vi "Receiver_Example - 2 Channel - Experiment_1.vi"() -> ()   [LabVIEW 2022 SP3]
panel:
  out "Constellation Map 4":cluster{"Constellation":cdb[]}[](graph)
  out "No. Bits LP 2":dbl
  in  "Expected message 2 HP 3":string="Critical Dataaaaa\nCritical Dataaaaa\nCritical Dataaaaa\nCritical Dataaaaa\nCritical Dataaaaa"
  out "Inst. BER HP 3":dbl format="%#_4g"
  out "Acum. Err HP 3":dbl
  out "Acc. BER  HP 3":dbl format="%#_4g"
  out "No. Bits HP 3":dbl
  in  "Boolean 5":bool
  out "Expected message  HP  Detected 3":string="Critical Dataaaaa\nCritical Dataaaaa\nCritical Dataaaaa\nCritical Dataaaaa\nCritical Dataaaaa"
  out "Constellation Map 3":cdb[](graph)
  out "Iterations 2":i32
  in  "OFDM - 4QAM/16QAM":bool
  in  "Tab Control 2":enum32{"OFDM - 4QAM", "16QAM"}(tab)
  in  "Tab Control":enum32{"USRP Parameters", "Rx Info", "BER"}(tab)
  in  "USRP ControledParameters":T1={"Active Antenna"="RX2", "Gain (dB)"=10.0, "Carrier Frequency"=2400000000.0, "IQ Rate"=2000000.0, "Active channels"="0,1"} {"IQ Rate" format="%#_6p"; "Carrier Frequency" format="%#_6p"; "Gain (dB)" format="%#_6f"}
  in  "Device selection":refnum<k15>="RIO0"
  in  "Trigger level":dbl=0.005 format="%f"
  out "?":T2
  out "SIG valid?":bool
  out "Frequency offset":dbl
  out "Coerced Parameters":T3={"IQ Rate"=100000.0, "Carrier  Freq."=100000.0, "Gain"=0.0} {"Gain" format="%#_6f"; "Carrier  Freq." format="%#_6p"; "IQ Rate" format="%#_6p"}
  out "Error out":errorcluster
  out "Frequency offset 3":dbl
  out "SIG valid? 3":bool
  out "Error out 2":errorcluster
  out "?":T2
  in  "Boolean":bool
  in  "Expected message LP":string="Non Critical Data\nNon Critical Data\nNon Critical Data\nNon Critical Data\nNon Critical Data"
  in  "Record BER":bool
  in  "Refresh Button":bool
  out "Inst. BER LP":dbl format="%#_4g"
  out "No. Bits LP":dbl
  out "Acum. Err LP":dbl
  out "Acc. BER LP":dbl format="%#_4g"
  in  "Expected message 2 HP":string="Critical Dataaaaa\nCritical Dataaaaa\nCritical Dataaaaa\nCritical Dataaaaa\nCritical Dataaaaa"
  out "Inst. BER HP":dbl format="%#_4g"
  out "Acum. Err HP":dbl
  out "No. Bits HP":dbl
  out "Acc. BER  HP":dbl format="%#_4g"
  out "Expected message LP Detected":string="Non Critical Data\nNon Critical Data\nNon Critical Data\nNon Critical Data\nNon Critical Data"
  out "Expected message  HP  Detected":string="Critical Dataaaaa\nCritical Dataaaaa\nCritical Dataaaaa\nCritical Dataaaaa\nCritical Dataaaaa"
  in  "Boolean 2":bool
  out "Constellation Map":cdb[](graph)
  out "Low-Power Decoded Message":string
  out "High-Power Decoded Message":string
  out "Low-Power BER Graph":dbl(graph)
  out "High-Power BER Graph":dbl(graph)
  out "Low-Power Instantaneous BER Graph":u8(slide) scale=0.0..100.0
  out "High-Power Instantaneous BER Graph":u8(slide) scale=0.0..100.0
  in  "Low-Power Window Size":dbl=15.0 format="%#_6p"
  in  "High-Power Window Size":dbl=15.0 format="%#_6p"
  out "Reconstructed Image":T4(plugin-control)
  out "High-Power Decoded Message 3":string
  in  "High-Power Window Size 3":dbl=15.0 format="%#_6p"
  out "High-Power Instantaneous BER Graph 3":u8(slide) scale=0.0..100.0
  out "High-Power BER Graph 3":dbl(graph)
  out "Expected message  HP  Detected 2":string="Critical Dataaaaa\nCritical Dataaaaa\nCritical Dataaaaa\nCritical Dataaaaa\nCritical Dataaaaa"
  in  "Boolean 3":bool
  in  "High-Power Window Size 2":dbl=15.0 format="%#_6p"
  out "High-Power Instantaneous BER Graph 2":u8(slide) scale=0.0..100.0
  out "High-Power BER Graph 2":dbl(graph)
  out "No. Bits HP 2":dbl
  out "Acc. BER  HP 2":dbl format="%#_4g"
  out "Acum. Err HP 2":dbl
  out "Inst. BER HP 2":dbl format="%#_4g"
  in  "Expected message 2 HP 2":string="Critical Dataaaaa\nCritical Dataaaaa\nCritical Dataaaaa\nCritical Dataaaaa\nCritical Dataaaaa"
  out "High-Power Decoded Message 2":string
  in  "Record BER 2":bool
  out "Constellation Map 2":cdb[](graph)
  out "Frequency offset 2":dbl
  out "SIG valid? 2":bool
  in  "Refresh Button 2":bool
  out "Reconstructed Image":T4(plugin-control)
  out "Iterations":i32
  in  "error in (no error)":errorcluster
  # "OFDM Superposition Coded Receiver"
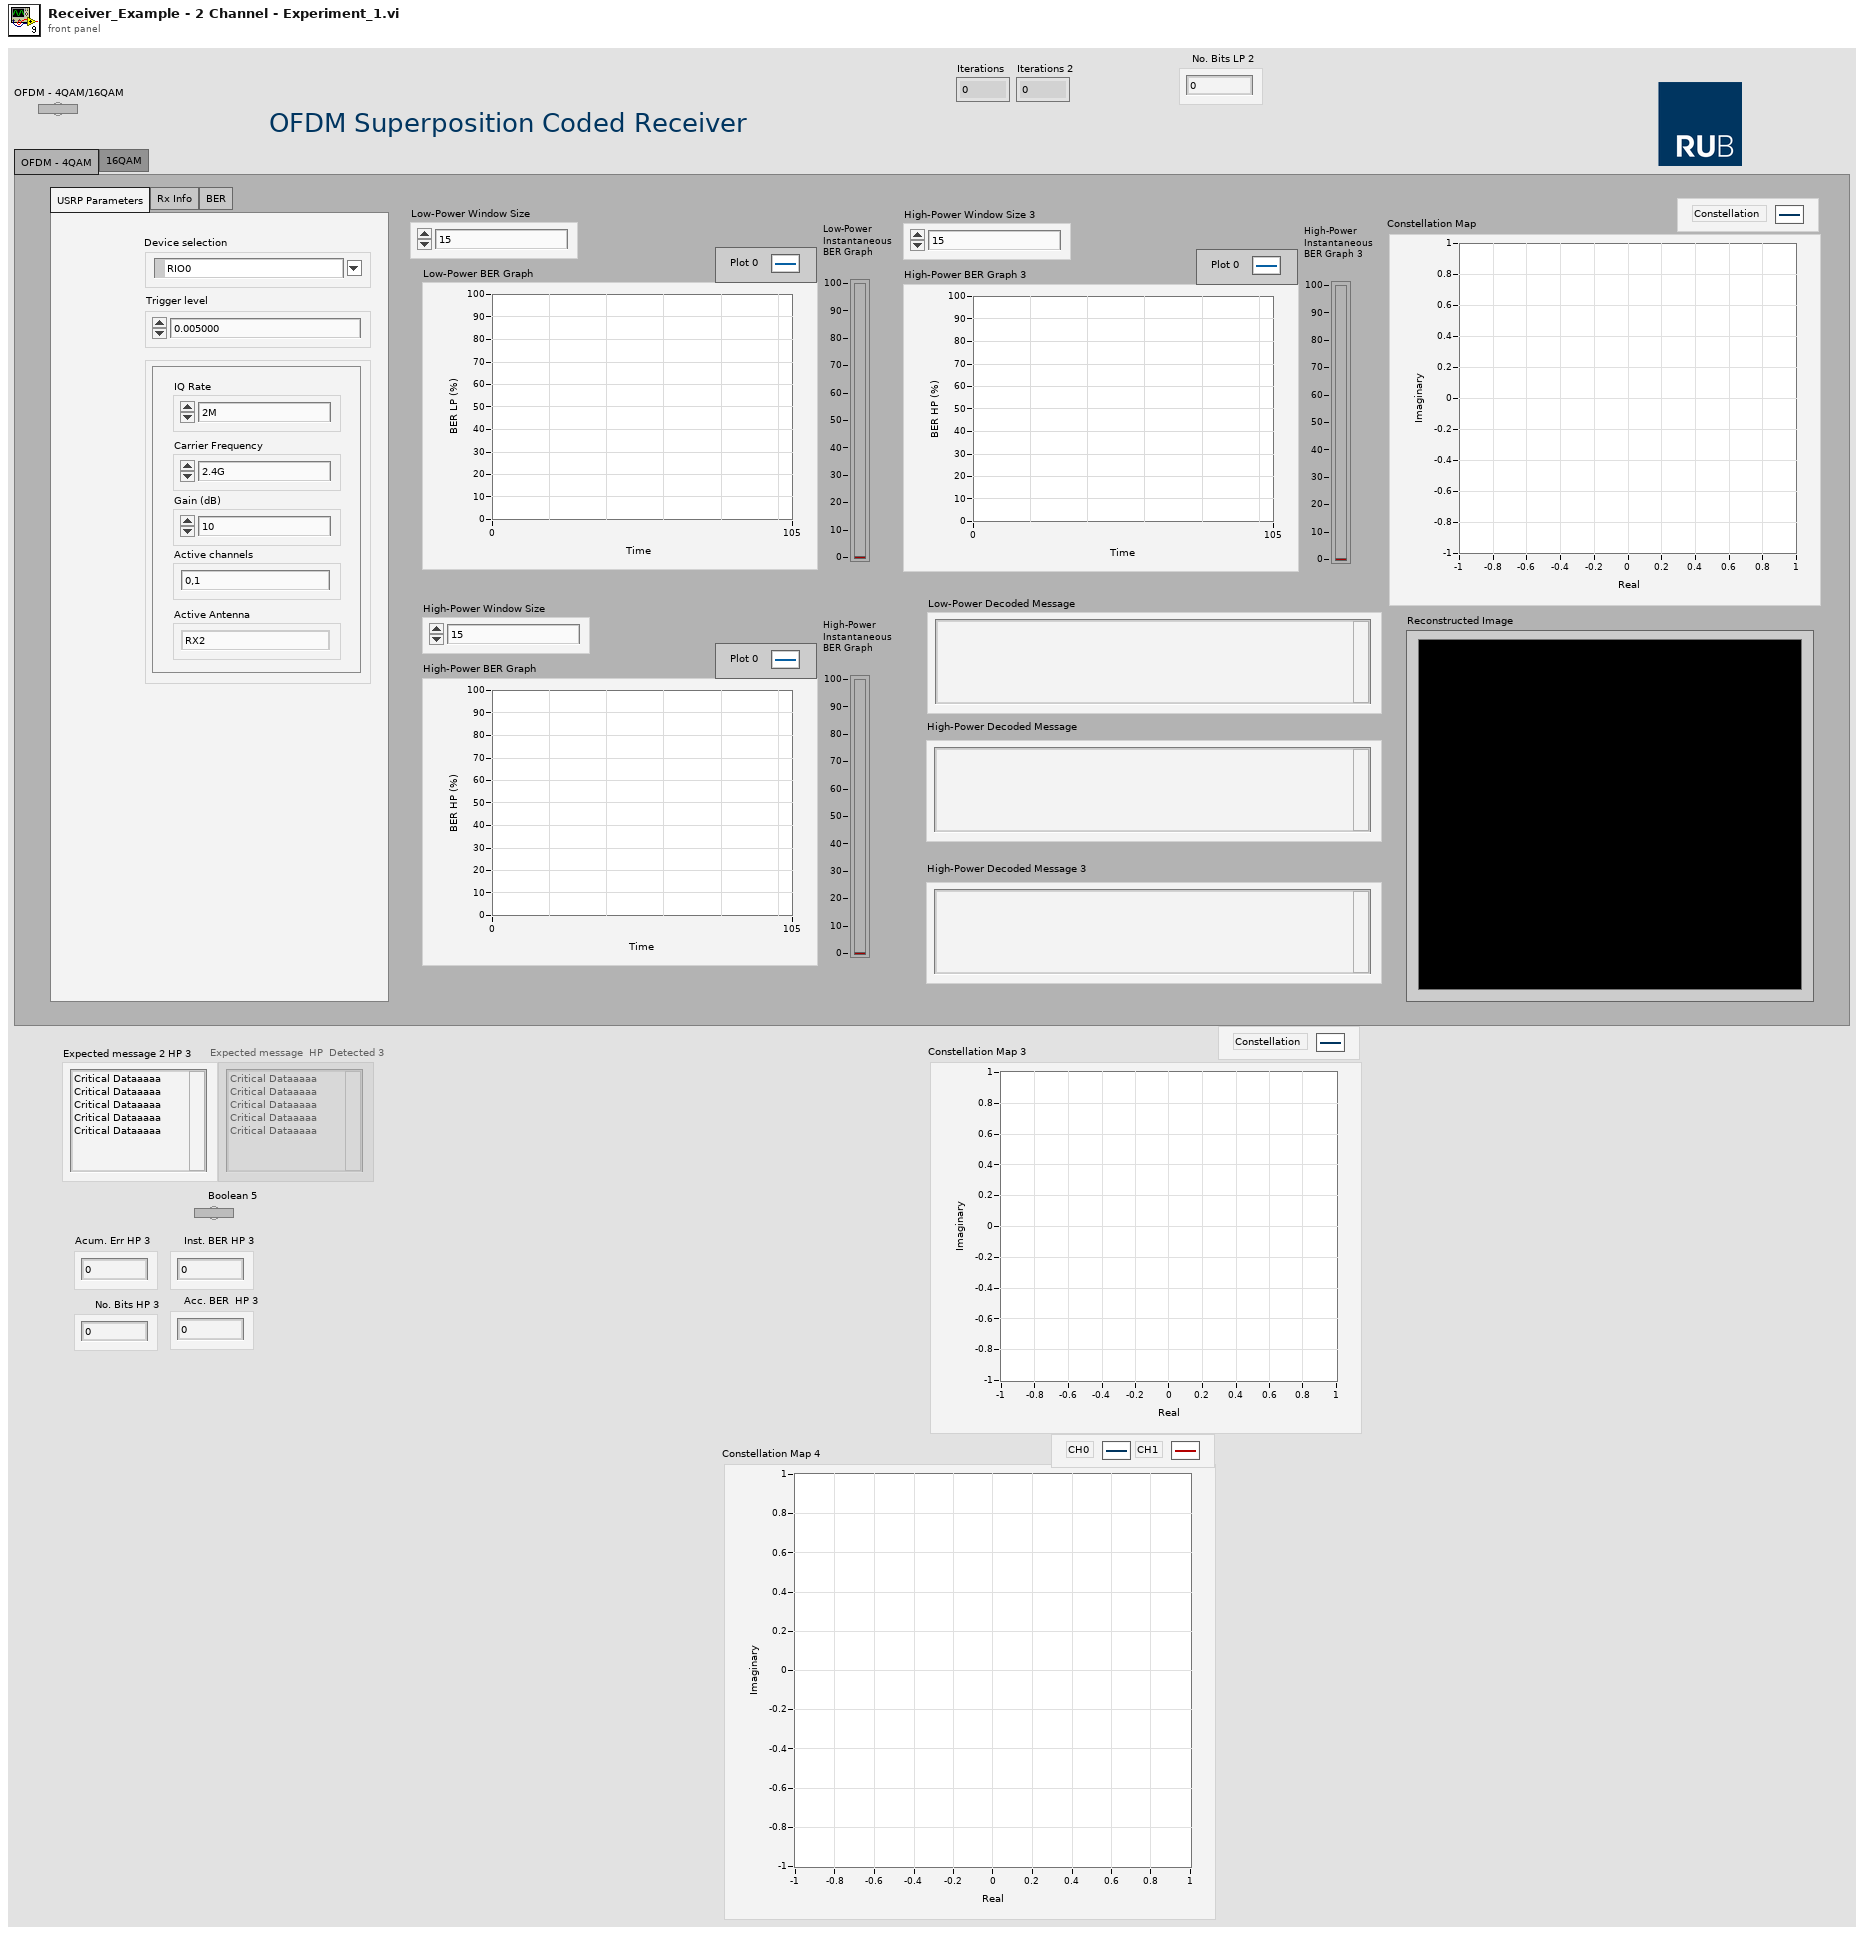
[diagram p1: front panel]
types:
  T1 = cluster{"Active Antenna":string, "Gain (dB)":dbl, "Carrier Frequency":dbl, "IQ Rate":dbl, "Active channels":string}
  T2 = cluster{"Modulation type":enum16{"QPSK(4QAM)", "64QAM", "16QAM", "BPSK"}, "BCC rate (k/n)":enum16{"1/2", "2/3", "3/4"}}
  T3 = cluster{"IQ Rate":dbl, "Carrier  Freq.":dbl, "Gain":dbl}
  T4 = typedef "IMAQ Image.ctl" = refnum<image>
  T5 = cluster{"coerced IQ rate":dbl, "coerced carrier frequency":dbl, "coerced gain":dbl}
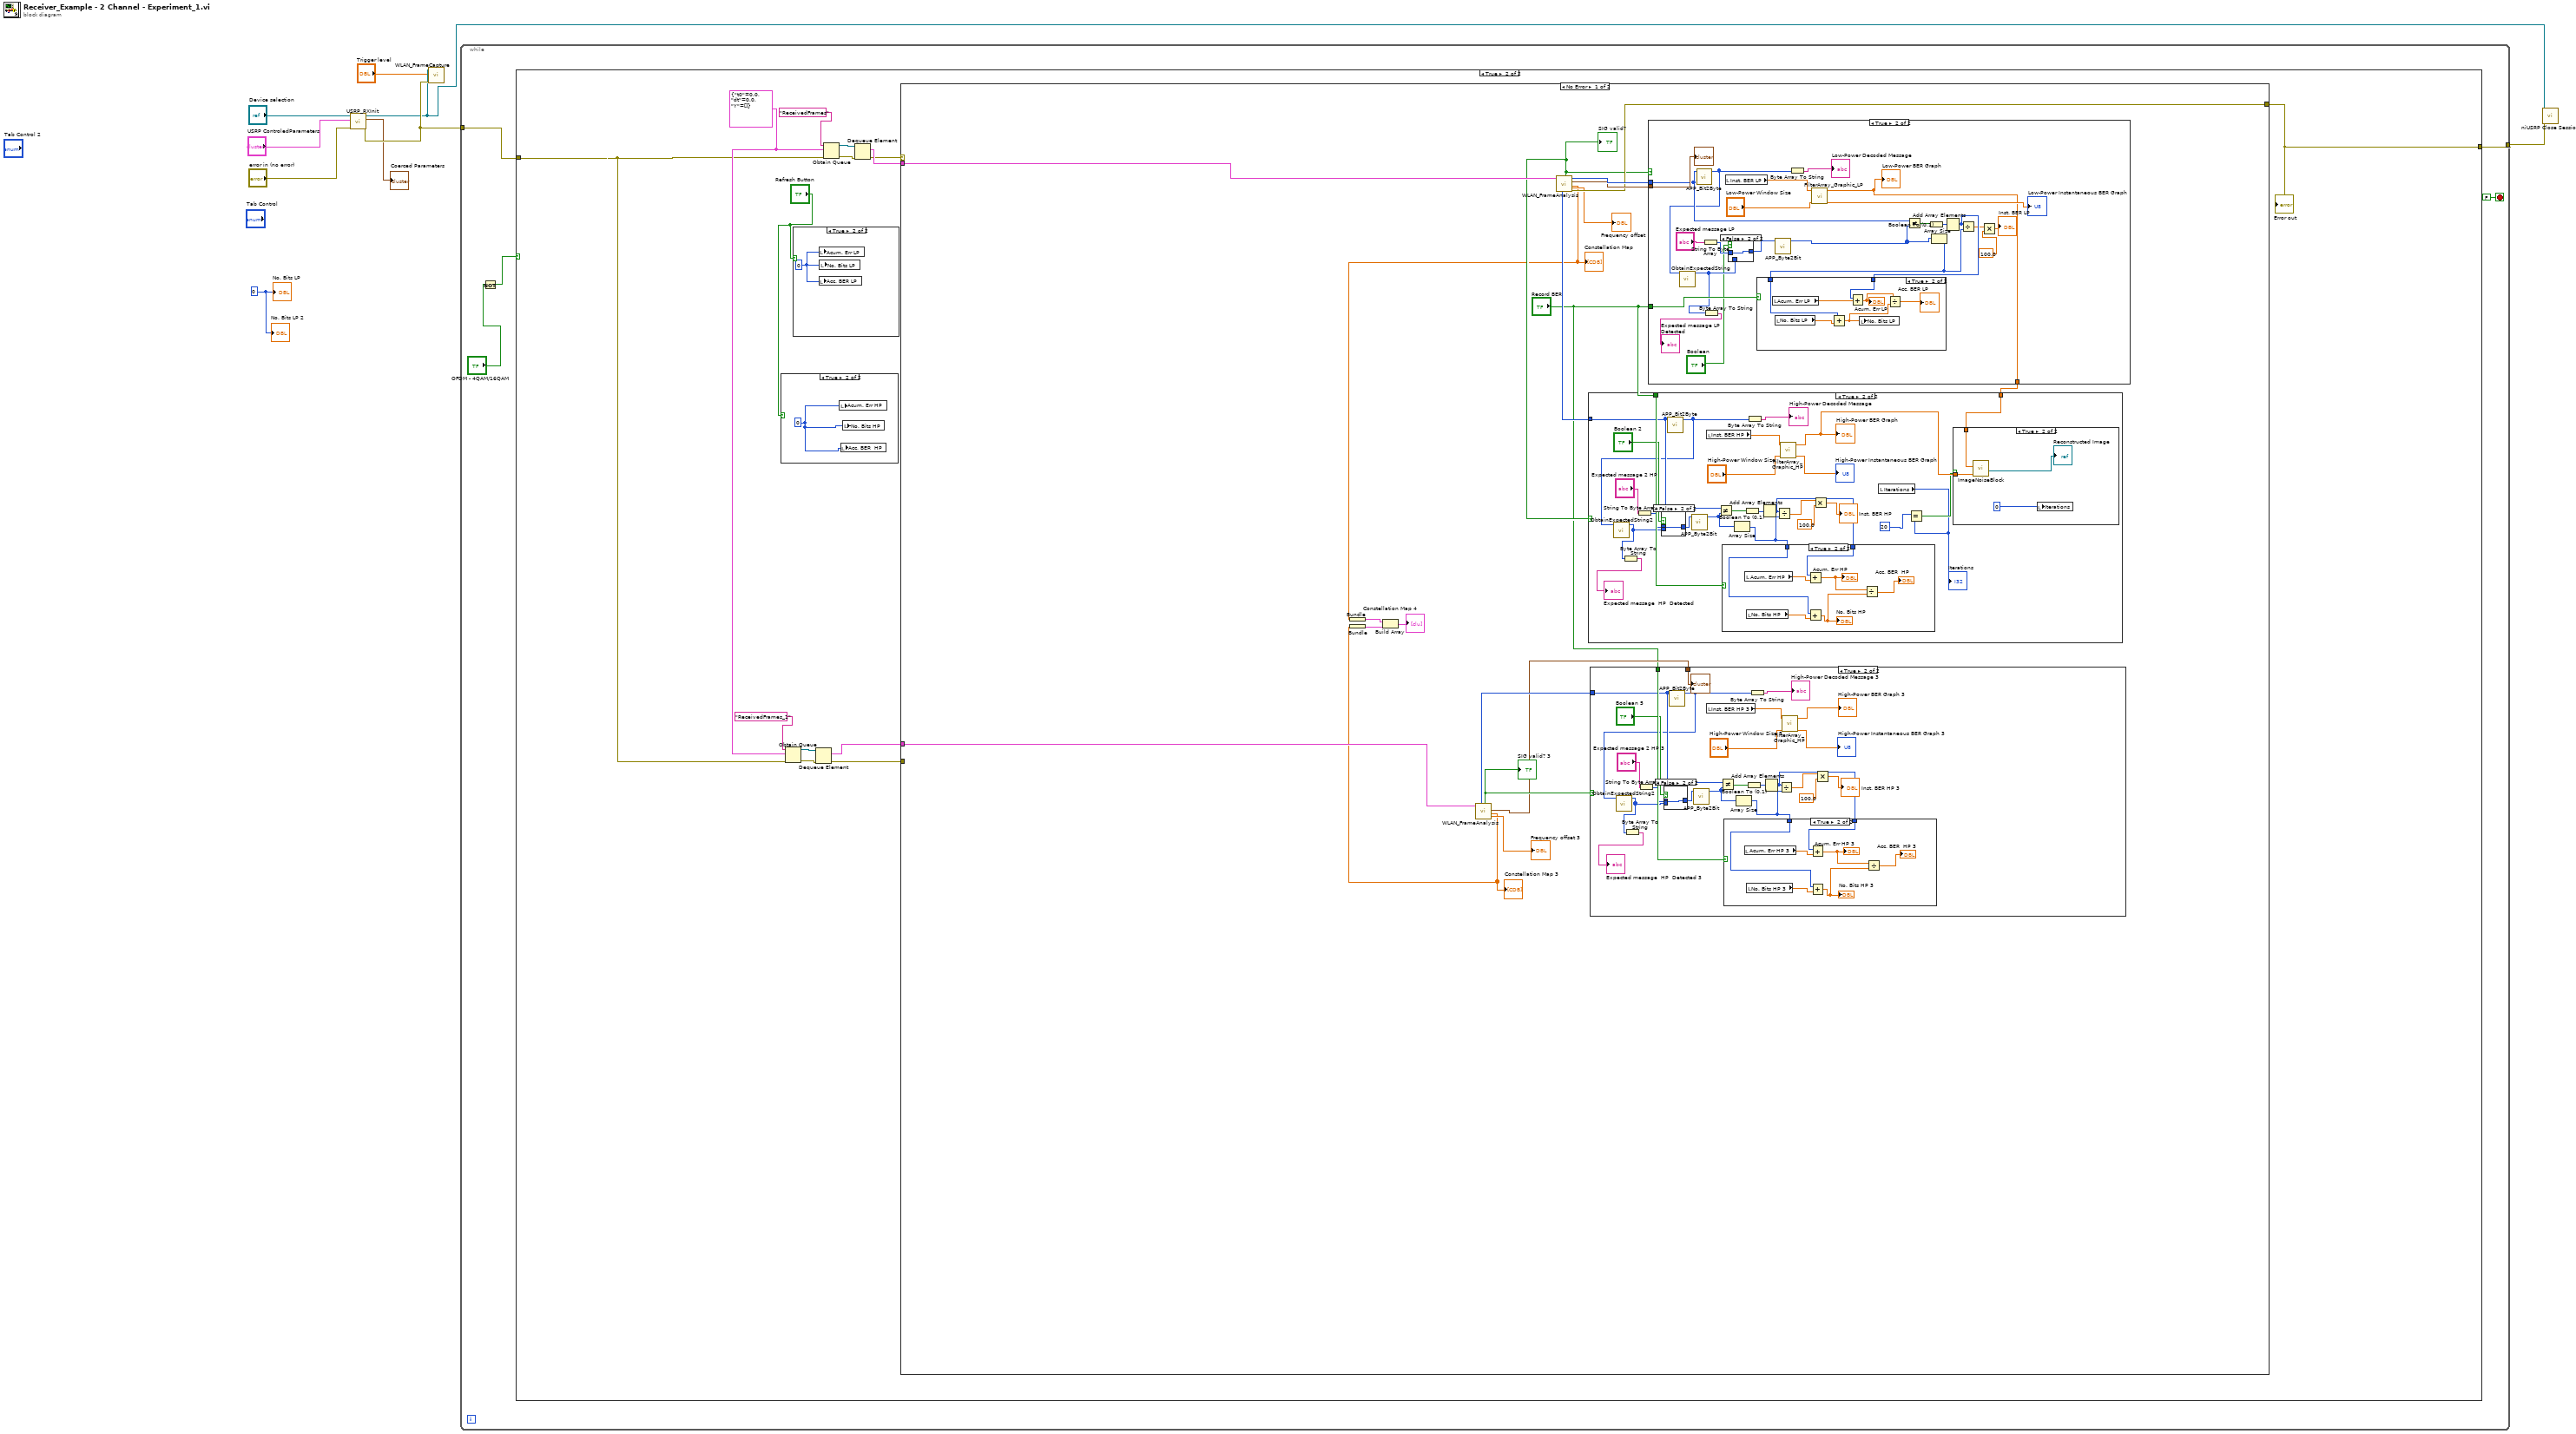
[diagram p0: block diagram]
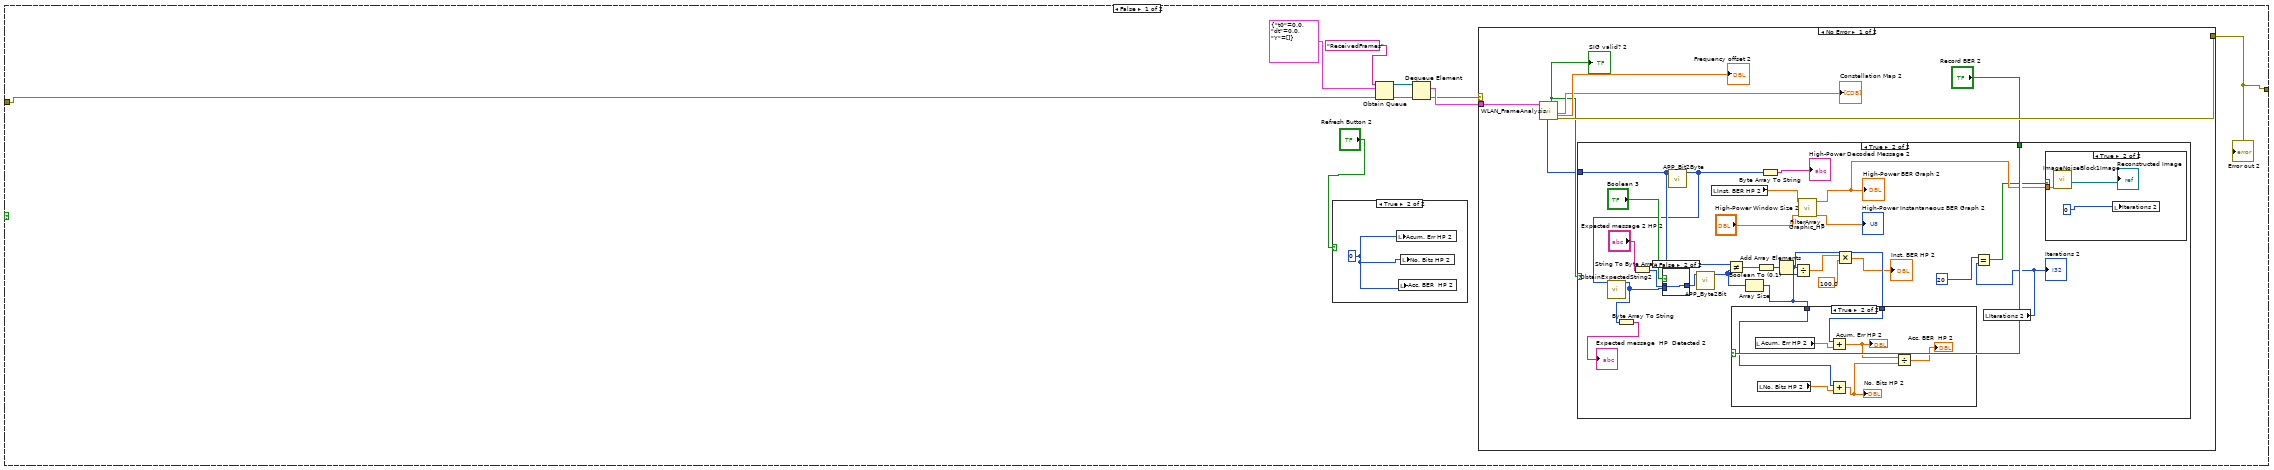
[diagram p2: hidden frame]
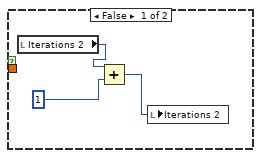
[diagram p5: hidden frame]
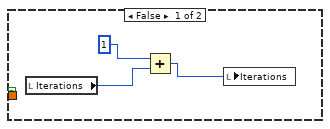
[diagram p16: hidden frame]
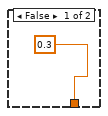
[diagram p18: hidden frame]
diagram:
  w1 = 0
  n1 = call "USRP_RXInit.vi"("device names"="Device selection", "USRP ControledParameters"="USRP ControledParameters", "error in (no error)"="error in (no error)") -> ("session handle out"=w6:refnum<k15>, "USRP CoercedParamters"=→"Coerced Parameters":T5, "error out"=w8:errorcluster)  [unwired: 5 in]
  n2 = call "WLAN_FrameCapture.vi"("error in (no error)"=w8, "Trigger level"="Trigger level", "session handle"=w6) -> ()  [unwired: 8 in]
  n3 = while {
    tunnel: w8 -> [w14]
    tunnel: [w13] -> w7
    stop <- FALSE stop-if-true
    n4 = Not(x="OFDM - 4QAM/16QAM") -> (.not. x?=w10:bool)
    n5 = case shown="True" w10 {
      tunnel: w14 -> [w16 w75]
      tunnel: [w15 w80] -> w13
      frame False {
        n6 = case shown="True" "Refresh Button 2" {
          frame False {
          }
          frame True {
            w24 = 0
            n7 = local write "Acum. Err HP 2"(w24) -> ()
            n8 = local write "Acc. BER  HP 2"(w24) -> ()
            n9 = local write "No. Bits HP 2"(w24) -> ()
          }
        }
        n10 = Obtain Queue(name (unnamed)="ReceivedFrames", element data type=cluster{"t0":dbl, "dt":dbl, "Y":cdb[]} {"t0"=0.0, "dt"=0.0, "Y"=[]} ("data"), error in (no error)=w16) -> (queue out=w17:refnum<queue>, error out=w20:errorcluster)  [unwired: 2 in, 1 out]
        n11 = Dequeue Element(queue=w17, error in (no error)=w20) -> (element=w19:cluster{"t0":dbl, "dt":dbl, "Y":cdb[]}, error out=w18:errorcluster)  [unwired: 1 in, 2 out]
        n12 = case shown="No Error" w18 {
          selector: w18 -> [_ w72]
          tunnel: w19 -> [w30 _]
          tunnel: [w31 w72] -> w15
          frame No Error {
            n13 = call "WLAN_FrameAnalysis.vi"("input cluster"=w30) -> ("error out"=w31:errorcluster, "Constellation"=→"Constellation Map 2":cdb[], "Frequency offset"=→"Frequency offset 2":dbl, "SIG valid?"=w26:bool, "outputbitsHP"=w25:i8[])  [unwired: 4 in, 2 out]
            "SIG valid? 2" <- w26
            n14 = case shown="True" w26 {
              tunnel: "Record BER 2" -> [_ w50]
              tunnel: w25 -> [_ w45]
              frame False {
              }
              frame True {
                n15 = String To Byte Array(string="Expected message 2 HP 2") -> (unsigned byte array=w43:u8[])
                n16 = call "APP_Bit2Byte.vi"("input bit stream"=w45) -> ("output byte stream"=w39:u8[])  [unwired: 10 in]
                n17 = call "ObtainExpectedString2.vi"("Array"=w39) -> ("detectedMessage"=w41:i8[])  [unwired: 9 in]
                n18 = Byte Array To String(unsigned byte array=w41) -> (string=→"Expected message  HP  Detected 2":string)
                n19 = case shown="False" "Boolean 3" {
                  tunnel: [w63 w64] -> w44
                  tunnel: w43 -> [_ w64]
                  tunnel: w41 -> [w63 _]
                  frame True {
                  }
                  frame False {
                  }
                }
                n20 = call "APP_Byte2Bit.vi"("input byte stream"=w44) -> ("output bit stream"=w46:i8[])  [unwired: 10 in]
                n21 = local read "Inst. BER HP 2"() -> (w49:dbl)
                n22 = Not Equal?(x=w45, y=w46) -> (x != y?=w54:bool[])
                n23 = Array Size(array=w46) -> (size(s)=w51:i32)
                n24 = Boolean To (0,1)(Boolean=w54) -> (0, 1=w53:i16[])
                n25 = Byte Array To String(unsigned byte array=w39) -> (string=→"High-Power Decoded Message 2":string)
                n26 = Add Array Elements(numeric array=w53) -> (sum=w52:i16)
                n27 = case shown="True" w50 {
                  tunnel: w52 -> [_ w70]
                  tunnel: w51 -> [_ w65]
                  frame False {
                  }
                  frame True {
                    n28 = local read "Acum. Err HP 2"() -> (w71:dbl)
                    n29 = local read "No. Bits HP 2"() -> (w67:dbl)
                    n30 = Add(x=w70, y=w71) -> (x+y=w69:dbl)
                    "Acum. Err HP 2" <- w69
                    n31 = Add(x=w65, y=w67) -> (x+y=w66:dbl)
                    "No. Bits HP 2" <- w66
                    n32 = Divide(x=w69, y=w66) -> (x/y=→"Acc. BER  HP 2":dbl)
                  }
                }
                n33 = Divide(x=w52, y=w51) -> (x/y=w38:dbl)
                n34 = call "FilterArray_Graphic_HP.vi"("Window Size"="High-Power Window Size 2", "Instantaneous BER"=w49) -> ("Slide Bar"=→"High-Power Instantaneous BER Graph 2":dbl, "Graph Instantaneous BER"=w35:dbl)  [unwired: 4 in]
                "High-Power BER Graph 2" <- w35
                n35 = Multiply(x=w38, y=100.0) -> (x*y=→"Inst. BER HP 2":dbl)
                n36 = local read "Iterations 2"() -> (w33:i32)
                "Iterations 2" <- w33
                n37 = Equal?(x=20, y=w33) -> (x = y?=w32:bool)
                n38 = case shown="True" w32 {
                  tunnel: w35 -> [_ w62]
                  frame False {
                    n39 = local read "Iterations 2"() -> (w59:i32)
                    n40 = Add(x=w59, y=1) -> (x+y=w57:i32)
                    n41 = local write "Iterations 2"(w57) -> ()
                  }
                  frame True {
                    n42 = call "ImageNoiseBlock1Image.vi"("BERHP"=w62) -> ("High-Power Image"=→"Reconstructed Image":T4)  [unwired: 9 in]
                    n43 = local write "Iterations 2"(0) -> ()
                  }
                }
              }
            }
          }
          frame Error {
          }
        }
        "Error out 2" <- w15
      }
      frame True {
        w76 = cluster{"t0":dbl, "dt":dbl, "Y":cdb[]} {"t0"=0.0, "dt"=0.0, "Y"=[]} ("data")
        n44 = case shown="True" "Refresh Button" {
          frame False {
          }
          frame True {
            w87 = 0
            n45 = local write "Acum. Err HP"(w87) -> ()
            n46 = local write "Acc. BER  HP"(w87) -> ()
            n47 = local write "No. Bits HP"(w87) -> ()
          }
        }
        n48 = Obtain Queue(name (unnamed)="ReceivedFrames_1", element data type=w76, error in (no error)=w75) -> (queue out=w77:refnum<queue>, error out=w78:errorcluster)  [unwired: 2 in, 1 out]
        n49 = case shown="True" "Refresh Button" {
          frame False {
          }
          frame True {
            w88 = 0
            n50 = local write "Acum. Err LP"(w88) -> ()
            n51 = local write "Acc. BER LP"(w88) -> ()
            n52 = local write "No. Bits LP"(w88) -> ()
          }
        }
        n53 = Dequeue Element(queue=w77, error in (no error)=w78) -> (element=w73:cluster{"t0":dbl, "dt":dbl, "Y":cdb[]}, error out=w74:errorcluster)  [unwired: 1 in, 2 out]
        n54 = Obtain Queue(name (unnamed)="ReceivedFrames", element data type=w76, error in (no error)=w75) -> (queue out=w81:refnum<queue>, error out=w84:errorcluster)  [unwired: 2 in, 1 out]
        n55 = Dequeue Element(queue=w81, error in (no error)=w84) -> (element=w83:cluster{"t0":dbl, "dt":dbl, "Y":cdb[]}, error out=w82:errorcluster)  [unwired: 1 in, 2 out]
        n56 = case shown="No Error" w82 {
          selector: w82 -> [_ w215]
          tunnel: w83 -> [w104 _]
          tunnel: [w105 w215] -> w80
          tunnel: w74 -> [_ _]
          tunnel: w73 -> [w96 _]
          frame No Error {
            n57 = call "WLAN_FrameAnalysis.vi"("input cluster"=w96) -> ("Constellation"=w90:cdb[], "Modulation parameter"=w95:T2, "Frequency offset"=→"Frequency offset 3":dbl, "SIG valid?"=w98:bool, "outputbitsHP"=w97:i8[])  [unwired: 4 in, 2 out]
            "SIG valid? 3" <- w98
            "Constellation Map 3" <- w90
            n58 = Bundle("Constellation"=w90) -> (w92:cluster{"Constellation":cdb[]})  [unwired: 1 in]
            n59 = call "WLAN_FrameAnalysis.vi"("input cluster"=w104) -> ("error out"=w105:errorcluster, "Constellation"=w89:cdb[], "Modulation parameter"=w106:T2, "output bits"=w107:i8[], "Frequency offset"=→"Frequency offset":dbl, "SIG valid?"=w102:bool, "outputbitsHP"=w101:i8[])  [unwired: 4 in]
            "SIG valid?" <- w102
            "Constellation Map" <- w89
            n60 = Bundle("Constellation"=w89) -> (w91:cluster{"Constellation":cdb[]})  [unwired: 1 in]
            n61 = Build Array(w91, w92) -> (→"Constellation Map 4":cluster{"Constellation":cdb[]}[])
            n62 = case shown="True" w98 {
              tunnel: "Record BER" -> [_ w124]
              tunnel: w97 -> [_ w118]
              tunnel: w95 -> [_ w108]
              frame False {
              }
              frame True {
                n63 = String To Byte Array(string="Expected message 2 HP 3") -> (unsigned byte array=w116:u8[])
                n64 = call "APP_Bit2Byte.vi"("input bit stream"=w118) -> ("output byte stream"=w112:u8[])  [unwired: 10 in]
                n65 = call "ObtainExpectedString2.vi"("Array"=w112) -> ("detectedMessage"=w114:i8[])  [unwired: 9 in]
                n66 = Byte Array To String(unsigned byte array=w114) -> (string=→"Expected message  HP  Detected 3":string)
                n67 = case shown="False" "Boolean 5" {
                  tunnel: [w131 w132] -> w117
                  tunnel: w116 -> [_ w132]
                  tunnel: w114 -> [w131 _]
                  frame True {
                  }
                  frame False {
                  }
                }
                n68 = call "APP_Byte2Bit.vi"("input byte stream"=w117) -> ("output bit stream"=w119:i8[])  [unwired: 10 in]
                n69 = local read "Inst. BER HP 3"() -> (w123:dbl)
                n70 = Not Equal?(x=w118, y=w119) -> (x != y?=w128:bool[])
                n71 = Array Size(array=w119) -> (size(s)=w125:i32)
                n72 = Boolean To (0,1)(Boolean=w128) -> (0, 1=w127:i16[])
                n73 = Byte Array To String(unsigned byte array=w112) -> (string=→"High-Power Decoded Message 3":string)
                n74 = Add Array Elements(numeric array=w127) -> (sum=w126:i16)
                n75 = case shown="True" w124 {
                  tunnel: w126 -> [_ w138]
                  tunnel: w125 -> [_ w133]
                  frame False {
                  }
                  frame True {
                    n76 = local read "Acum. Err HP 3"() -> (w139:dbl)
                    n77 = local read "No. Bits HP 3"() -> (w135:dbl)
                    n78 = Add(x=w138, y=w139) -> (x+y=w137:dbl)
                    "Acum. Err HP 3" <- w137
                    n79 = Add(x=w133, y=w135) -> (x+y=w134:dbl)
                    "No. Bits HP 3" <- w134
                    n80 = Divide(x=w137, y=w134) -> (x/y=→"Acc. BER  HP 3":dbl)
                  }
                }
                n81 = Divide(x=w126, y=w125) -> (x/y=w111:dbl)
                n82 = call "FilterArray_Graphic_HP.vi"("Window Size"="High-Power Window Size 3", "Instantaneous BER"=w123) -> ("Slide Bar"=→"High-Power Instantaneous BER Graph 3":dbl, "Graph Instantaneous BER"=→"High-Power BER Graph 3":dbl)  [unwired: 4 in]
                n83 = Multiply(x=w111, y=100.0) -> (x*y=→"Inst. BER HP 3":dbl)
                "?" <- w108
              }
            }
            n84 = case shown="True" w102 {
              tunnel: w107 -> [_ w190]
              tunnel: w106 -> [_ w205]
              tunnel: "Record BER" -> [_ w199]
              tunnel: [0.3 ("Graph Instantaneous BER") w195] -> w100
              frame False {
              }
              frame True {
                n85 = call "APP_Bit2Byte.vi"("input bit stream"=w190) -> ("output byte stream"=w186:u8[])  [unwired: 10 in]
                n86 = call "ObtainExpectedString.vi"("Array"=w186) -> ("detectedMessage"=w188:i8[])  [unwired: 9 in]
                n87 = String To Byte Array(string="Expected message LP") -> (unsigned byte array=w191:u8[])
                n88 = Byte Array To String(unsigned byte array=w188) -> (string=→"Expected message LP Detected":string)
                n89 = local read "Inst. BER LP"() -> (w198:dbl)
                n90 = case shown="False" "Boolean" {
                  tunnel: [w206 w207] -> w192
                  tunnel: w191 -> [_ w207]
                  tunnel: w188 -> [w206 _]
                  frame True {
                  }
                  frame False {
                  }
                }
                n91 = call "APP_Byte2Bit.vi"("input byte stream"=w192) -> ("output bit stream"=w193:i8[])  [unwired: 10 in]
                n92 = Byte Array To String(unsigned byte array=w186) -> (string=→"Low-Power Decoded Message":string)
                n93 = call "FilterArray_Graphic_LP.vi"("Window Size"="Low-Power Window Size", "Instantaneous BER"=w198) -> ("Slide Bar"=→"Low-Power Instantaneous BER Graph":dbl, "Graph Instantaneous BER"=w195:dbl)  [unwired: 4 in]
                "Low-Power BER Graph" <- w195
                n94 = Not Equal?(x=w190, y=w193) -> (x != y?=w201:bool[])
                n95 = Boolean To (0,1)(Boolean=w201) -> (0, 1=w194:i16[])
                n96 = Array Size(array=w193) -> (size(s)=w203:i32)
                n97 = Add Array Elements(numeric array=w194) -> (sum=w200:i16)
                n98 = case shown="True" w199 {
                  tunnel: w203 -> [_ w213]
                  tunnel: w200 -> [_ w211]
                  frame False {
                  }
                  frame True {
                    n99 = local read "Acum. Err LP"() -> (w212:dbl)
                    n100 = local read "No. Bits LP"() -> (w214:dbl)
                    n101 = Add(x=w213, y=w214) -> (x+y=w208:dbl)
                    n102 = Add(x=w211, y=w212) -> (x+y=w210:dbl)
                    "Acum. Err LP" <- w210
                    n103 = local write "No. Bits LP"(w208) -> ()
                    n104 = Divide(x=w210, y=w208) -> (x/y=→"Acc. BER LP":dbl)
                  }
                }
                n105 = Divide(x=w200, y=w203) -> (x/y=w185:dbl)
                n106 = Multiply(x=w185, y=100.0) -> (x*y=→"Inst. BER LP":dbl)
                "?" <- w205
              }
            }
            n107 = case shown="True" w102 {
              tunnel: "Record BER" -> [_ w159]
              tunnel: w101 -> [_ w149]
              tunnel: w100 -> [_ w154]
              frame False {
              }
              frame True {
                n108 = String To Byte Array(string="Expected message 2 HP") -> (unsigned byte array=w147:u8[])
                n109 = call "APP_Bit2Byte.vi"("input bit stream"=w149) -> ("output byte stream"=w143:u8[])  [unwired: 10 in]
                n110 = call "ObtainExpectedString2.vi"("Array"=w143) -> ("detectedMessage"=w145:i8[])  [unwired: 9 in]
                n111 = Byte Array To String(unsigned byte array=w145) -> (string=→"Expected message  HP  Detected":string)
                n112 = case shown="False" "Boolean 2" {
                  tunnel: [w166 w167] -> w148
                  tunnel: w147 -> [_ w167]
                  tunnel: w145 -> [w166 _]
                  frame True {
                  }
                  frame False {
                  }
                }
                n113 = call "APP_Byte2Bit.vi"("input byte stream"=w148) -> ("output bit stream"=w153:i8[])  [unwired: 10 in]
                n114 = local read "Inst. BER HP"() -> (w158:dbl)
                n115 = Not Equal?(x=w149, y=w153) -> (x != y?=w163:bool[])
                n116 = Array Size(array=w153) -> (size(s)=w160:i32)
                n117 = Boolean To (0,1)(Boolean=w163) -> (0, 1=w162:i16[])
                n118 = Byte Array To String(unsigned byte array=w143) -> (string=→"High-Power Decoded Message":string)
                n119 = Add Array Elements(numeric array=w162) -> (sum=w161:i16)
                n120 = case shown="True" w159 {
                  tunnel: w161 -> [_ w180]
                  tunnel: w160 -> [_ w175]
                  frame False {
                  }
                  frame True {
                    n121 = local read "Acum. Err HP"() -> (w181:dbl)
                    n122 = local read "No. Bits HP"() -> (w177:dbl)
                    n123 = Add(x=w180, y=w181) -> (x+y=w179:dbl)
                    "Acum. Err HP" <- w179
                    n124 = Add(x=w175, y=w177) -> (x+y=w176:dbl)
                    "No. Bits HP" <- w176
                    n125 = Divide(x=w179, y=w176) -> (x/y=→"Acc. BER  HP":dbl)
                  }
                }
                n126 = Divide(x=w161, y=w160) -> (x/y=w142:dbl)
                n127 = call "FilterArray_Graphic_HP.vi"("Window Size"="High-Power Window Size", "Instantaneous BER"=w158) -> ("Slide Bar"=→"High-Power Instantaneous BER Graph":dbl, "Graph Instantaneous BER"=w155:dbl)  [unwired: 4 in]
                "High-Power BER Graph" <- w155
                n128 = Multiply(x=w142, y=100.0) -> (x*y=→"Inst. BER HP":dbl)
                n129 = local read "Iterations"() -> (w151:i32)
                "Iterations" <- w151
                n130 = Equal?(x=20, y=w151) -> (x = y?=w152:bool)
                n131 = case shown="True" w152 {
                  tunnel: w155 -> [_ w174]
                  tunnel: w154 -> [_ w173]
                  frame False {
                    n132 = local read "Iterations"() -> (w168:i32)
                    n133 = Add(x=1, y=w168) -> (x+y=w169:i32)
                    n134 = local write "Iterations"(w169) -> ()
                  }
                  frame True {
                    n135 = call "ImageNoiseBlock.vi"("BERLP"=w173, "BERHP"=w174) -> ("High-Power Image"=→"Reconstructed Image":T4)  [unwired: 8 in]
                    n136 = local write "Iterations"(0) -> ()
                  }
                }
              }
            }
          }
          frame Error {
          }
        }
        "Error out" <- w80
      }
    }
  }
  n137 = call <instrlib>:"niUSRP Close Session.vi"("session handle"=w6, "error in (no error)"=w7) -> ()  [unwired: 13 in, 1 out]
  "No. Bits LP" <- w1
  "No. Bits LP 2" <- w1
